vi "roller_getInputs.vi"(11 "Joysticks":T2) -> (3 "Roller Inputs":T1)   [LabVIEW 2013]
uses:
  roller_inputs.ctl
  util/joystick_vals.ctl
  <vilib>/Rock Robotics/WPI/Joystick/WPI_JoystickButtonState.ctl
panel:
  in  "Roller Inputs 2":T1
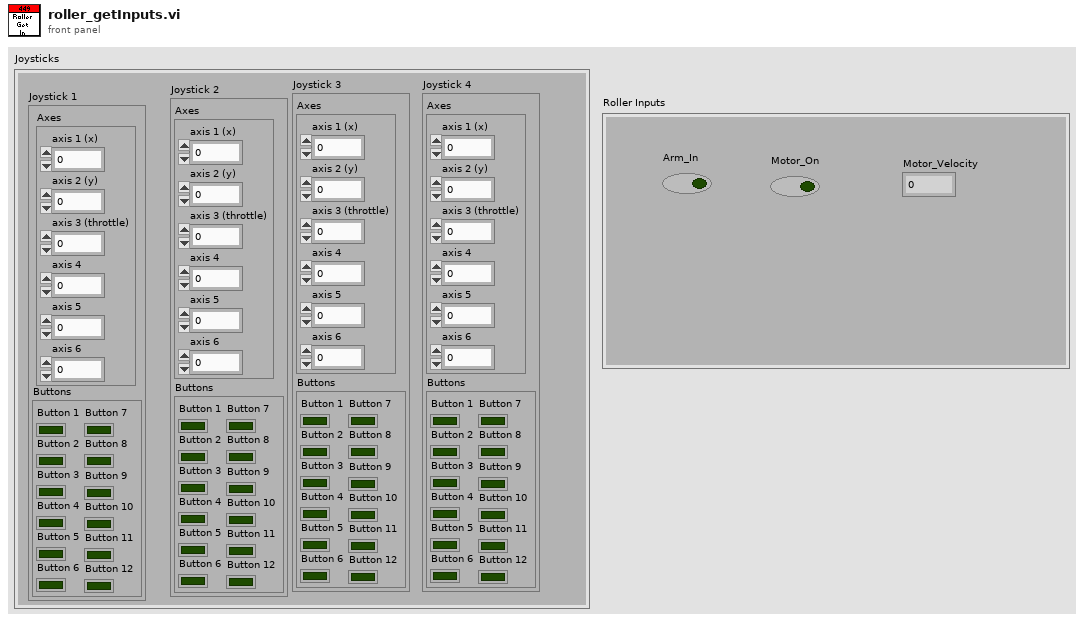
[diagram p1: front panel]
types:
  T1 = typedef "roller_inputs.ctl" = cluster{"Arm_In":bool, "Motor_On":bool, "Motor_Velocity":dbl}
  T2 = typedef "joystick_vals.ctl" = cluster{"Joystick 1":cluster{"Axes":cluster{"axis 1 (x)":dbl, "axis 2 (y)":dbl, "axis 3 (throttle)":dbl, "axis 4":dbl, "axis 5":dbl, "axis 6":dbl}, "Buttons":T3}, "Joystick 2":cluster{"Axes":cluster{"axis 1 (x)":dbl, "axis 2 (y)":dbl, "axis 3 (throttle)":dbl, "axis 4":dbl, "axis 5":dbl, "axis 6":dbl}, "Buttons":T3}, "Joystick 3":cluster{"Axes":cluster{"axis 1 (x)":dbl, "axis 2 (y)":dbl, "axis 3 (throttle)":dbl, "axis 4":dbl, "axis 5":dbl, "axis 6":dbl}, "Buttons":T3}, "Joystick 4":cluster{"Axes":cluster{"axis 1 (x)":dbl, "axis 2 (y)":dbl, "axis 3 (throttle)":dbl, "axis 4":dbl, "axis 5":dbl, "axis 6":dbl}, "Buttons":T3}}
  T3 = typedef "WPI_JoystickButtonState.ctl" = cluster{"Button 1":bool, "Button 2":bool, "Button 3":bool, "Button 4":bool, "Button 5":bool, "Button 6":bool, "Button 7":bool, "Button 8":bool, "Button 9":bool, "Button 10":bool, "Button 11":bool, "Button 12":bool}
  T4 = cluster{"Axes":cluster{"axis 1 (x)":dbl, "axis 2 (y)":dbl, "axis 3 (throttle)":dbl, "axis 4":dbl, "axis 5":dbl, "axis 6":dbl}, "Buttons":T3}
  T5 = cluster{"axis 1 (x)":dbl, "axis 2 (y)":dbl, "axis 3 (throttle)":dbl, "axis 4":dbl, "axis 5":dbl, "axis 6":dbl}
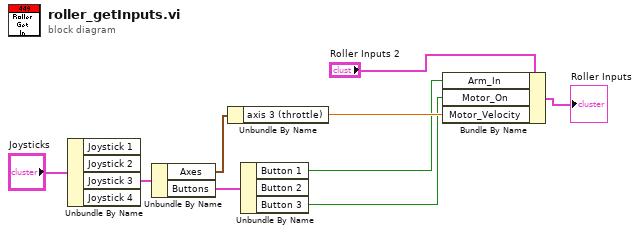
[diagram p0: block diagram]
diagram:
  n1 = Unbundle By Name("Joysticks") -> ("Joystick 3"=w7:T4)  [unwired: 3 out]
  n2 = Unbundle By Name(w7) -> ("Axes"=w6:T5, "Buttons"=w4:T3)
  n3 = Unbundle By Name(w6) -> ("axis 3 (throttle)"=w5:dbl)
  n4 = Unbundle By Name(w4) -> ("Button 1"=w2:bool, "Button 3"=w1:bool)  [unwired: 1 out]
  n5 = Bundle By Name(cluster="Roller Inputs 2", "Arm_In"=w2, "Motor_On"=w1, "Motor_Velocity"=w5) -> (→"Roller Inputs":T1)
